vi "9048_main.vi"() -> ()   [LabVIEW 2023]
uses:
  JSON Command.ctl
  Action.ctl
  <vilib>/FPGAPlugInAG/cRIO-9048/niLvFpga_Open_cRIO-9048.vi
  <vilib>/rvi/interface/common/dynamic/niFpgaDynamicAddResources.vi
  <vilib>/Utility/error.llb/Error Cluster From Error Code.vi
  <vilib>/rvi/errors/niLvFpgaAdjustHostInterfaceError.vi
  <vilib>/rvi/interface/common/niFpgaWaitOnOcc.vi
  <vilib>/FPGAPlugInAG/Dynamic/niLvFpga_Run_Dynamic.vi
  <vilib>/FPGAPlugInAG/Dynamic/niLvFpga_Close_Dynamic.vi
  <vilib>/rvi/interface/nirviOpenFPGA/nirviOpenFPGA.xnode
  FPGA Bitfiles/cryosimcontrolsy_FPGATarget_targetmainmem_OolXwFFypuY.lvbitx
  target_main_mem.vi
  <vilib>/rvi/interface/nirviReadWriteControl/nirviReadWriteControl.xnode
  <vilib>/rvi/interface/nirviMethod/nirviMethod.xnode
  <vilib>/rvi/interface/nirviCloseFPGA/nirviCloseFPGA.xnode
  <vilib>/FPGAPlugInAG/Dynamic/niLvFpga_ConfigureFifo_Dynamic.vi
  <vilib>/rvi/errors/niLvFpgaMergeErrorWithErrorCode.vi
  <vilib>/FPGAPlugInAG/Dynamic/niLvFpga_WriteFifo_Dynamic.vi
  NiFpgaLv.dll
  <vilib>/rvi/interface/Simulation/niFpgaSimulationCallBeginRW.vi
  <vilib>/FPGAPlugInAG/Dynamic/niLvFpga_ReadFifo_Dynamic.vi
  <vilib>/FPGAPlugInAG/Dynamic/niLvFpga_StopFifo_Dynamic.vi
  LabView workspace/CoboltLaserDriver.lvlib
panel:
  in  "Stop VI":bool
  out "FPGA VI Reference Out":refnum<k20>
  out "Abort":bool
  out "remote port":u16
  out "remote address":string
  in  "Send PORT":u16=7704
  out "From Client:":string
  out "RAW JSON":T1
  out "ACK sent":string
  in  "FPGA Status Update Loop Time (uSec)":u32=1000
  out "UDP Sent":string
  in  "Event":string
  in  "FPGA Status":string
  in  "Receive PORT":u16=7705
  in  "UDP Address (IP)":string="169.254.31.168"
  out "Digitals":u8
  out "Analogue Line 2":u8
  out "Analogue Line 1":u8
  out "Analogue Line 0":u8
  out "408 Violet Toggle":bool
  in  "Analogue Line 6":u32=20
  out "Laser Port":refnum<visa-resource-name>
  out "Laser Response OK":bool=TRUE
  out "488 Blue Toggle":bool
  out "532 Red Toggle":bool
  out "638 Green Toggle":bool
  in  "Analogue Line 5":u32=20
  in  "Analogue Line 4":u32=20
  in  "Analogue Line 3":u32=20
  in  "Digitals Action Table":T2[](array[typedef])
  in  "Analogue 2 Action Table":T2[](array[typedef])
  in  "Analogue 1 Action Table":T2[](array[typedef])
  in  "Analogue 0 Action Table":T2[](array[typedef])
  out "Tick Ref":u32
  out "Addr Digitals":u32
  out "repDuration (ms)":u64
  out "numReps":u64
  out "From sendStartStopIndexes":u64[](array[numeric])
  out "Addr Analogue 1":u32
  out "Addr Analogue 2":u32
  out "Addr Analogue 0":u32
  in  "att 6":fxp<+/-,20,5> format="%#.3f"
  in  "att 7":fxp<+/-,20,5> format="%#.3f"
  in  "att 5":fxp<+/-,20,5> format="%#.3f"
  in  "att 4":fxp<+/-,20,5> format="%#.3f"
  in  "att 3":fxp<+/-,20,5> format="%#.3f"
  in  "att 2":fxp<+/-,20,5> format="%#.3f"
  in  "att 1":fxp<+/-,20,5> format="%#.3f"
  in  "Vps 5":fxp<+/-,20,5>
  in  "Vps 4":fxp<+/-,20,5>
  in  "Vps 2":fxp<+/-,20,5>
  in  "Vps 6":fxp<+/-,20,5>
  in  "Vps 3":fxp<+/-,20,5>
  in  "Vps 1":fxp<+/-,20,5>
  # "TCP Communication"
  # "UDP Communication"
  # "FPGA: Angle, Phase, and Color"
  # "FPGA: Laser On/Off and Power Control"
  # "Action Tables & Experiment Logging"
  # "Experiment Execution Trace"
  # "FPGA: Direct Set Analogue 1"
  # "FPGA: Direct Set Analogue 2"
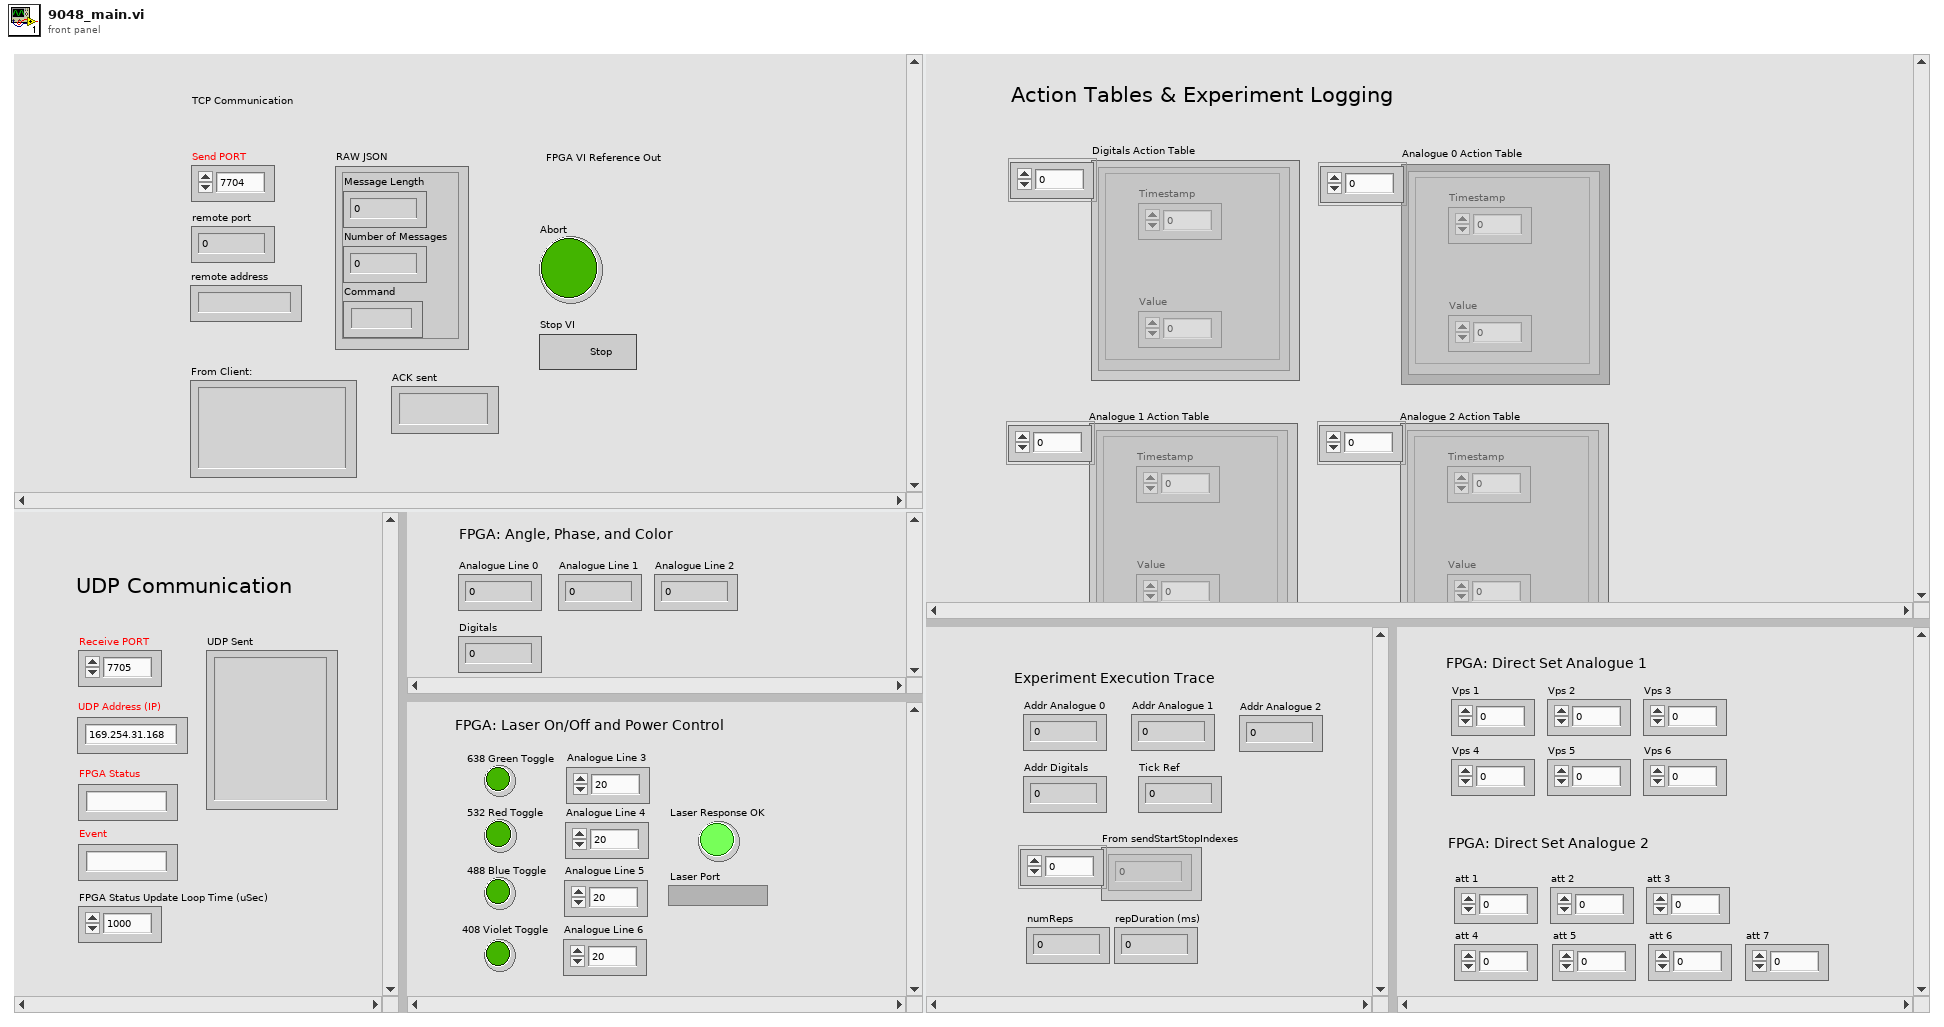
[diagram p1: front panel]
types:
  T1 = typedef "JSON Command.ctl" = cluster{"Message Length":i32, "Number of Messages":i32, "Command":string}
  T2 = typedef "Action.ctl" = cluster{"Timestamp":u32, "Value":u32}
  T3 = cluster{"Digital 0":bool, "Digital 1":bool, "Digital 2":bool}
  T4 = cluster{"Digitals":u8, "Analogue 0":u8, "Analogue 1":u8, "Event":string, "Analogue 2":u8, "Analogue 3":u32, "Analogue 4":u32, "Analogue 5":u32, "Analogue 6":u32}
  T5 = enum16{"Standard", "Buffered", "CRLF", "Immediate"}
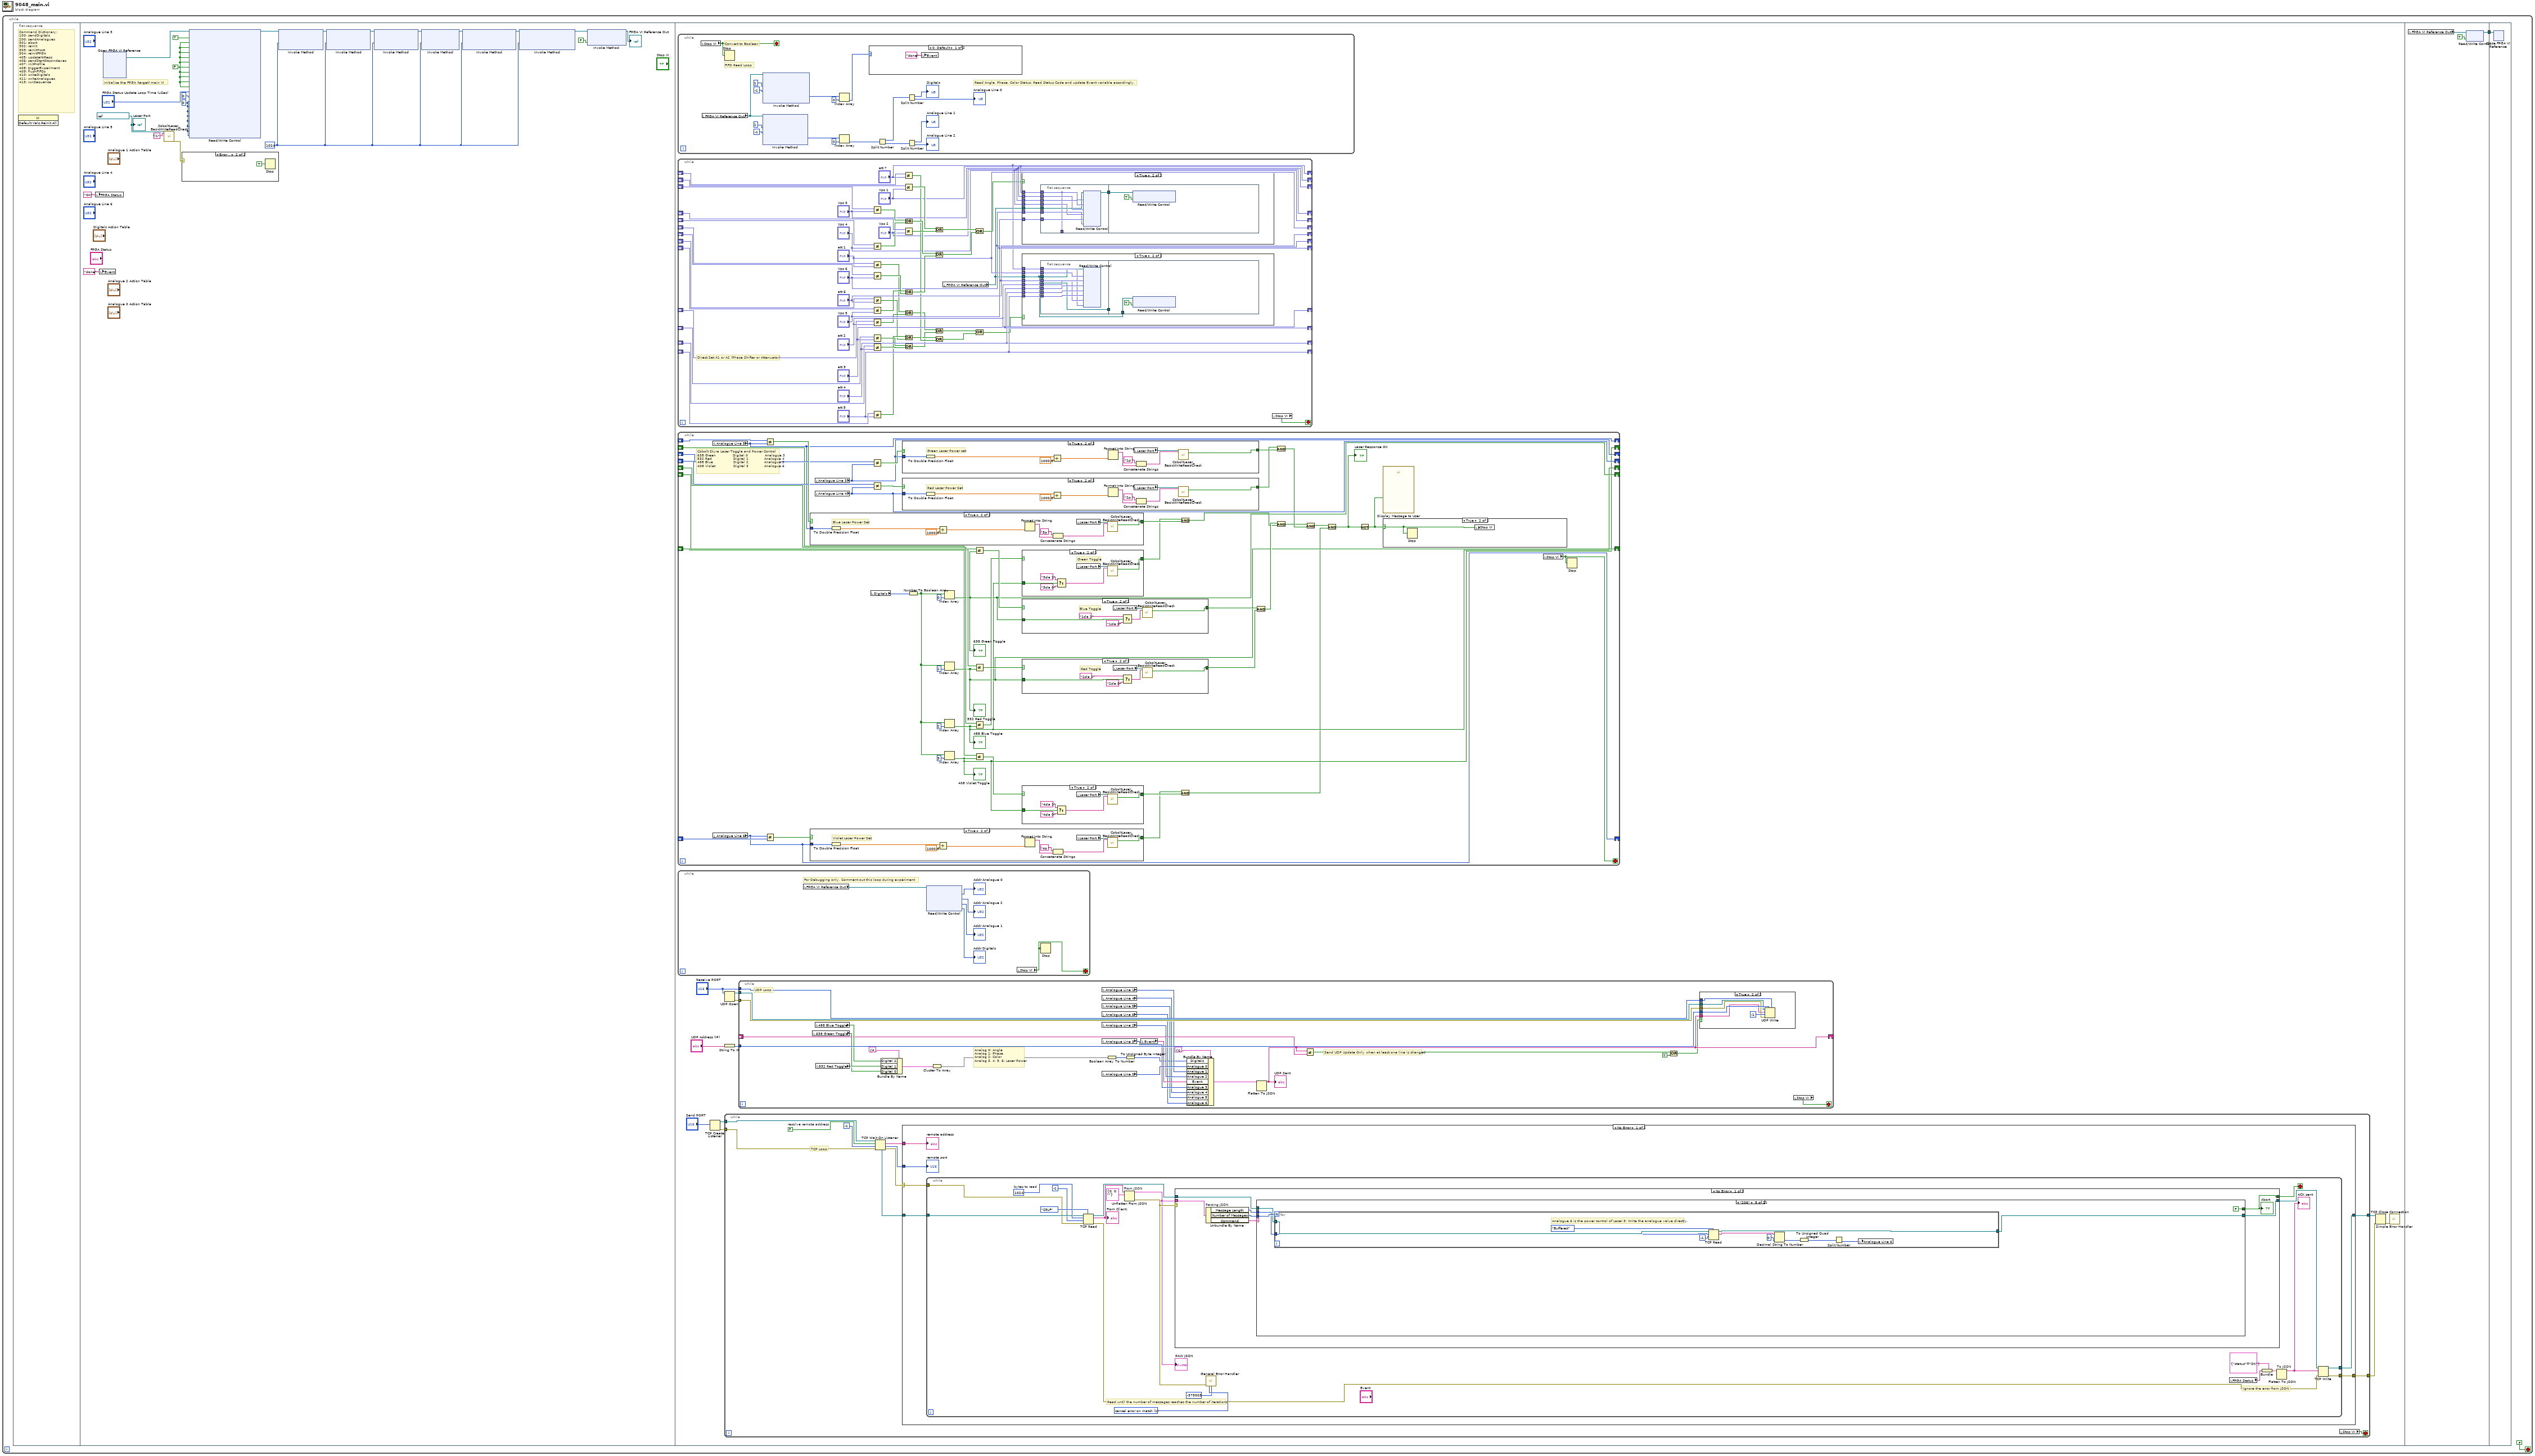
[diagram p0: block diagram]
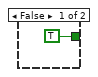
[diagram p5: hidden frame]
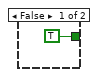
[diagram p6: hidden frame]
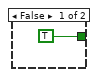
[diagram p8: hidden frame]
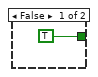
[diagram p9: hidden frame]
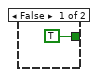
[diagram p10: hidden frame]
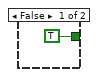
[diagram p11: hidden frame]
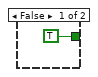
[diagram p12: hidden frame]
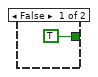
[diagram p13: hidden frame]
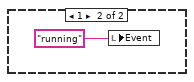
[diagram p14: hidden frame]
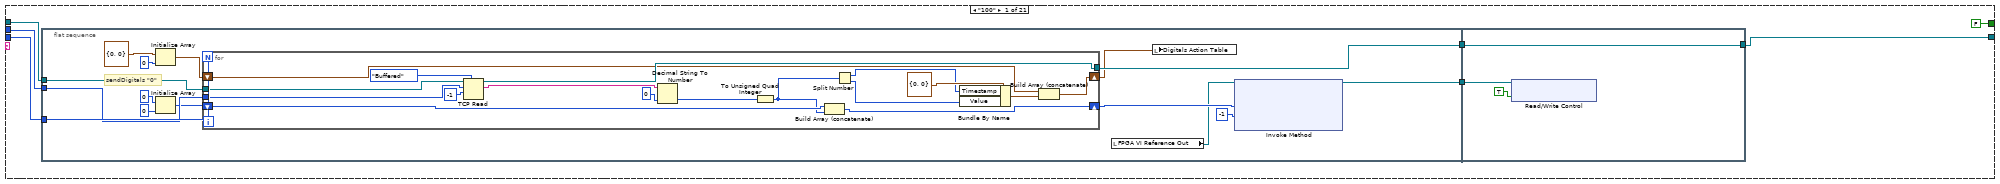
[diagram p16: hidden frame]
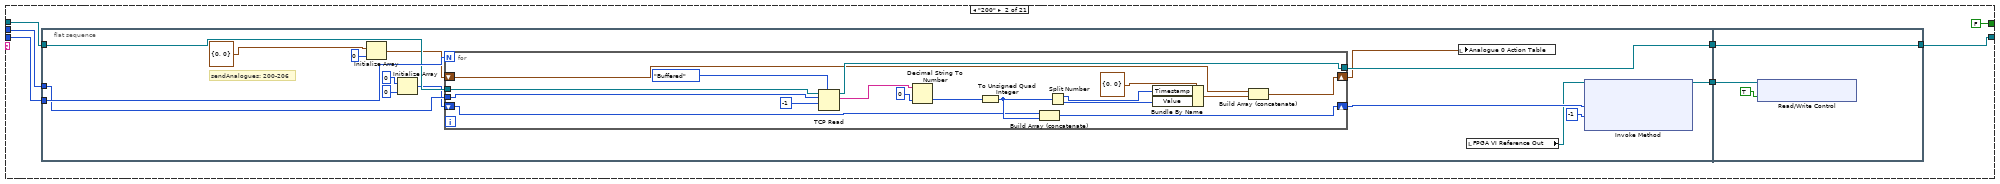
[diagram p17: hidden frame]
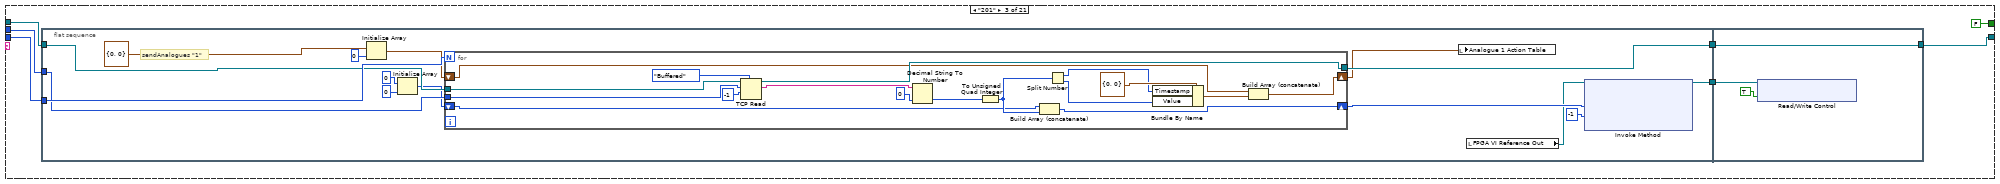
[diagram p18: hidden frame]
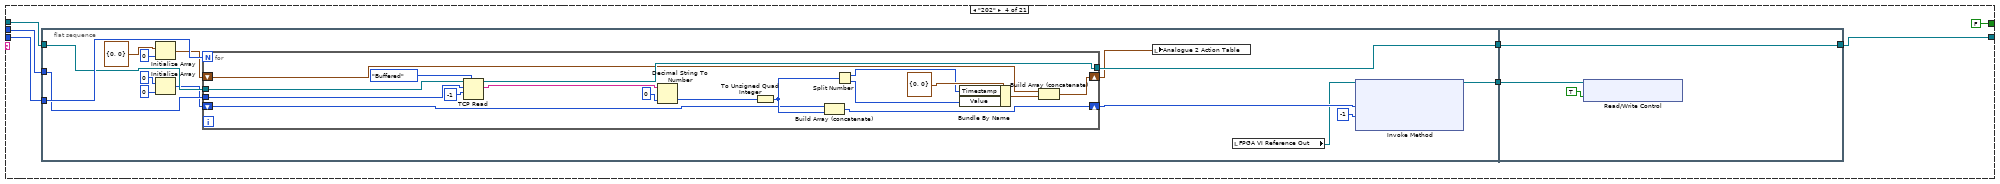
[diagram p19: hidden frame]
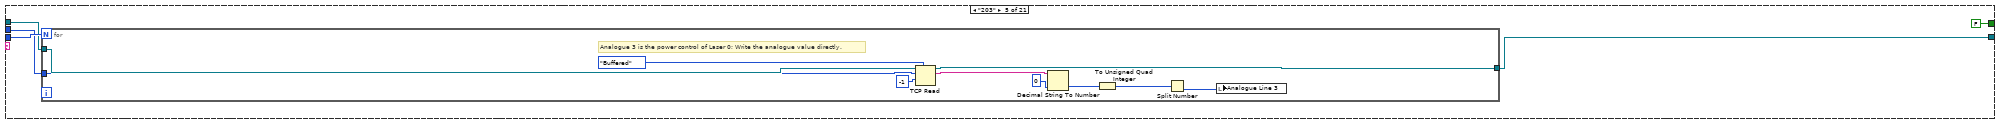
[diagram p20: hidden frame]
diagram:
  n1 = while {
    stop <- FALSE stop-if-true
    n2 = flat-sequence {
      tunnel: [w765] -> w2
      tunnel: w2 -> [w767]
      frame #0 {
        # "Command Dictionary:\n100: sendDigitals\n200: sendAnalogues\n301: abort\n302: reInit\n303: reInitHost\n304: reInitFPGA\n405: updateNrReps\n406: sendStartStopIndexes\n407: initProfile\n408: triggerExperiment\n409: flushFIFOs\n410: writeDigitals\n411: writeAnalogues\n413: runSequence"
        n3 = invoke class="VI" method="Default Vals.Reinit All"() -> ()  [unwired: 3 in, 3 out]
      }
      frame #1 {
        w3 = refnum<visa-resource-name> "ASRL3::INSTR" ("ComPort")
        w9 = u32 0 ("Addr Analogue 0")
        w8 = u32 1024 ("Requested Depth")
        w6 = FALSE ("Action Abort")
        # "Initialize the FPGA (target) main VI"
        n4 = local write "FPGA Status"("OK") -> ()
        n5 = local write "Event"("done") -> ()
        n6 = xnode "Open FPGA VI Reference"() -> ("FPGA VI Reference Out"=w12:refnum<k20>)  [unwired: 2 in, 1 out]
        n7 = call "CoboltLaser_BasicWriteReadCheck.vi"("ComPort"=w3, "Command"="l1") -> ("error out"=w4:errorcluster)  [unwired: 22 in, 3 out]
        n8 = case shown="Error .." w4 {
          frame No Error {
          }
          frame Error {
            n9 = Stop(stop? (T)=TRUE) -> ()
          }
        }
        n10 = xnode "Read/Write Control"("FPGA VI Reference In"=w12, "FPGA Tick Reset"=TRUE, "Abort"=w6, "Load Actions Analogue 0"=w6, "Load Actions Analogue 1"=w6, "Load Actions Analogue 2"=w6, "Load Actions Digitals"=w6, "Flush FIFO"=w6, "Trigger Experiment"=w6, "Set Analogue 0"=w6, "Set Analogue 1"=w6, "Set Analogue 2"=w6, "FPGA Status Update Loop Time (uSec)"="FPGA Status Update Loop Time (uSec)", "Status Code"=u8 0, "Addr Analogue 0"=w9, "Addr Analogue 1"=w9, "Addr Analogue 2"=w9, "Num of Actions Analogue 0"=w9, "Num of Actions Analogue 1"=w9, "Num of Actions Analogue 2"=w9, "Num of Actions Digitals"=w9, "Digitals"=w9) -> ("FPGA VI Reference Out"=w11:refnum<k20>)  [unwired: 1 in, 1 out]
        n11 = xnode "Invoke Method"("FPGA VI Reference In"=w11, "Requested Depth"=w8) -> ("FPGA VI Reference Out"=w22:refnum<k20>)  [unwired: 1 in, 2 out]
        n12 = xnode "Invoke Method"("FPGA VI Reference In"=w22, "Requested Depth"=w8) -> ("FPGA VI Reference Out"=w13:refnum<k20>)  [unwired: 1 in, 2 out]
        n13 = xnode "Invoke Method"("FPGA VI Reference In"=w13, "Requested Depth"=w8) -> ("FPGA VI Reference Out"=w21:refnum<k20>)  [unwired: 1 in, 2 out]
        n14 = xnode "Invoke Method"("FPGA VI Reference In"=w21, "Requested Depth"=w8) -> ("FPGA VI Reference Out"=w20:refnum<k20>)  [unwired: 1 in, 2 out]
        n15 = xnode "Invoke Method"("FPGA VI Reference In"=w20, "Requested Depth"=w8) -> ("FPGA VI Reference Out"=w19:refnum<k20>)  [unwired: 1 in, 2 out]
        n16 = xnode "Invoke Method"("FPGA VI Reference In"=w19, "Requested Depth"=w8) -> ("FPGA VI Reference Out"=w10:refnum<k20>)  [unwired: 1 in, 2 out]
        n17 = xnode "Invoke Method"("FPGA VI Reference In"=w10, "Wait Until Done (F)"=FALSE) -> ("FPGA VI Reference Out"=→"FPGA VI Reference Out":refnum<k20>)  [unwired: 1 in, 1 out]
        "Laser Port" <- w3
      }
      frame #2 {
        n18 = while {
          stop <- w248 stop-if-true
          # "Read Angle, Phase, Color Status; Read Status Code and update Event variable accordingly."
          # "FIFO Read Loop"
          # "Convert to Boolean"
          n19 = local read "Stop VI"() -> (w248:bool)
          n20 = local read "FPGA VI Reference Out"() -> (w249:refnum<k20>)
          n21 = Stop(stop? (T)=w248) -> ()
          n22 = xnode "Invoke Method"("FPGA VI Reference In"=w249, "Number of Elements"=u32 1, "Timeout (ms)"=-1) -> ("Data"=w253:u8[])  [unwired: 1 in, 3 out]
          n23 = xnode "Invoke Method"("FPGA VI Reference In"=w249, "Number of Elements"=u32 1, "Timeout (ms)"=-1) -> ("Data"=w262:u32[])  [unwired: 1 in, 3 out]
          n24 = Index Array(array=w253, index=0) -> (element=w254:u8)
          n25 = Index Array(array=w262, index=0) -> (element=w260:u32)
          n26 = case shown="0, Default" w254 {
            frame 0, Default {
              n27 = local write "Event"("done") -> ()
            }
            frame 1 {
              n28 = local write "Event"("running") -> ()
            }
          }
          n29 = Split Number(x=w260) -> (hi(x)=w259:u16, lo(x)=w258:u16)
          n30 = Split Number(x=w259) -> (hi(x)=→"Digitals":u8, lo(x)=→"Analogue Line 0":u8)
          n31 = Split Number(x=w258) -> (hi(x)=→"Analogue Line 1":u8, lo(x)=→"Analogue Line 2":u8)
        }
        n32 = while {
          shift-right: ["Vps 3"] -> _
          shift-left: _ -> [w85]
          shift-right: ["Vps 4"] -> _
          shift-left: _ -> [w84]
          shift-right: ["Vps 2"] -> _
          shift-left: _ -> [w86]
          shift-right: ["Vps 6"] -> _
          shift-left: _ -> [w82]
          shift-right: ["Vps 5"] -> _
          shift-left: _ -> [w83]
          shift-right: ["Vps 1"] -> _
          shift-left: _ -> [w87]
          shift-right: ["att 1"] -> _
          shift-left: _ -> [w67]
          shift-right: ["att 2"] -> _
          shift-left: _ -> [w66]
          shift-right: ["att 3"] -> _
          shift-left: _ -> [w65]
          shift-right: ["att 4"] -> _
          shift-left: _ -> [w64]
          shift-right: ["att 5"] -> _
          shift-left: _ -> [w63]
          shift-right: ["att 6"] -> _
          shift-left: _ -> [w62]
          shift-right: ["att 7"] -> _
          shift-left: _ -> [w61]
          stop <- w39 stop-if-true
          # "Direct Set A1 or A2 (Phase Shifter or Attenuator)"
          n33 = Not Equal?(x=w85, y="Vps 3") -> (x != y?=w79:bool)
          n34 = Not Equal?(x=w84, y="Vps 4") -> (x != y?=w78:bool)
          n35 = Not Equal?(x=w67, y="att 1") -> (x != y?=w53:bool)
          n36 = Not Equal?(x=w82, y="Vps 6") -> (x != y?=w76:bool)
          n37 = Not Equal?(x=w62, y="att 6") -> (x != y?=w48:bool)
          n38 = Not Equal?(x=w83, y="Vps 5") -> (x != y?=w77:bool)
          n39 = Not Equal?(x=w66, y="att 2") -> (x != y?=w52:bool)
          n40 = Not Equal?(x=w65, y="att 3") -> (x != y?=w51:bool)
          n41 = Not Equal?(x=w64, y="att 4") -> (x != y?=w50:bool)
          n42 = Not Equal?(x=w63, y="att 5") -> (x != y?=w49:bool)
          n43 = Not Equal?(x=w61, y="att 7") -> (x != y?=w47:bool)
          n44 = Not Equal?(x=w87, y="Vps 1") -> (x != y?=w81:bool)
          n45 = Or(x=w79, y=w78) -> (x .or. y?=w74:bool)
          n46 = Not Equal?(x=w86, y="Vps 2") -> (x != y?=w80:bool)
          n47 = Or(x=w77, y=w76) -> (x .or. y?=w73:bool)
          n48 = Or(x=w53, y=w52) -> (x .or. y?=w45:bool)
          n49 = Or(x=w49, y=w48) -> (x .or. y?=w46:bool)
          n50 = Or(x=w51, y=w50) -> (x .or. y?=w44:bool)
          n51 = Or(x=w81, y=w80) -> (x .or. y?=w75:bool)
          n52 = Or(x=w74, y=w73) -> (x .or. y?=w72:bool)
          n53 = Or(x=w45, y=w44) -> (x .or. y?=w42:bool)
          n54 = Or(x=w46, y=w47) -> (x .or. y?=w43:bool)
          n55 = local read "FPGA VI Reference Out"() -> (w40:refnum<k20>)
          n56 = Or(x=w75, y=w72) -> (x .or. y?=w36:bool)
          n57 = Or(x=w42, y=w43) -> (x .or. y?=w41:bool)
          n58 = case shown="True" w36 {
            tunnel: w40 -> [_ w109]
            tunnel: "Vps 1" -> [_ w108]
            tunnel: "Vps 2" -> [_ w114]
            tunnel: "Vps 3" -> [_ w113]
            tunnel: "Vps 4" -> [_ w112]
            tunnel: "Vps 5" -> [_ w111]
            tunnel: "Vps 6" -> [_ w110]
            frame False {
            }
            frame True {
              n59 = flat-sequence {
                tunnel: w109 -> [w117]
                tunnel: w110 -> [w118]
                tunnel: w111 -> [w119]
                tunnel: w112 -> [w120]
                tunnel: w113 -> [w121]
                tunnel: w114 -> [w122]
                tunnel: w108 -> [w115]
                tunnel: [w116] -> w107
                tunnel: [w115] -> _
                tunnel: w107 -> [w123]
                frame #0 {
                  n60 = xnode "Read/Write Control"("FPGA VI Reference In"=w117, "Vps1"=w115, "Vps2"=w122, "Vps3"=w121, "Vps4"=w120, "Vps5"=w119, "Vps6"=w118) -> ("FPGA VI Reference Out"=w116:refnum<k20>)  [unwired: 1 in, 1 out]
                }
                frame #1 {
                  n61 = xnode "Read/Write Control"("FPGA VI Reference In"=w123, "Direct Set Analogue 1"=TRUE) -> ()  [unwired: 1 in, 2 out]
                }
              }
            }
          }
          n62 = case shown="True" w41 {
            tunnel: "att 2" -> [_ w95]
            tunnel: "att 1" -> [_ w96]
            tunnel: "att 3" -> [_ w94]
            tunnel: "att 4" -> [_ w93]
            tunnel: "att 5" -> [_ w92]
            tunnel: "att 6" -> [_ w91]
            tunnel: "att 7" -> [_ w90]
            tunnel: w40 -> [_ w88]
            frame False {
            }
            frame True {
              n63 = flat-sequence {
                tunnel: w88 -> [w97]
                tunnel: w90 -> [w98]
                tunnel: w91 -> [w99]
                tunnel: w92 -> [w100]
                tunnel: w93 -> [w101]
                tunnel: w94 -> [w102]
                tunnel: w95 -> [w103]
                tunnel: w96 -> [w104]
                tunnel: [w97] -> w89
                tunnel: w89 -> [_]
                tunnel: w88 -> [w106]
                frame #0 {
                  n64 = xnode "Read/Write Control"("FPGA VI Reference In"=w97, "att1"=w104, "att2"=w103, "att3"=w102, "att4"=w101, "att5"=w100, "att6"=w99, "att7"=w98) -> ()  [unwired: 1 in, 2 out]
                }
                frame #1 {
                  n65 = xnode "Read/Write Control"("FPGA VI Reference In"=w106, "Direct Set Analogue 2"=TRUE) -> ()  [unwired: 1 in, 2 out]
                }
              }
            }
          }
          n66 = local read "Stop VI"() -> (w39:bool)
        }
        n67 = while {
          shift-right: [w141] -> _
          shift-left: _ -> [w171]
          shift-right: [w139] -> _
          shift-left: _ -> [w166]
          shift-right: [w138] -> _
          shift-left: _ -> [w167]
          shift-right: [w159] -> _
          shift-left: _ -> [w162]
          shift-right: [w158] -> _
          shift-left: _ -> [w161]
          shift-right: [w157] -> _
          shift-left: _ -> [w160]
          shift-right: [w132] -> _
          shift-left: _ -> [w135]
          shift-right: [w129] -> _
          shift-left: _ -> [w131]
          stop <- w146 stop-if-true
          # "Cobolt Skyra Laser Toggle and Power Control\n638 Green               Digital 0               Analogue 3\n532 Red                   Digital 1              Analogue 4\n488 Blue                  Digital 2              Analogue 5\n408 Violet                Digital 3              Analogue 6"
          n68 = local read "Analogue Line 5"() -> (w159:u32)
          n69 = local read "Analogue Line 6"() -> (w129:u32)
          n70 = Not Equal?(x=w162, y=w159) -> (x != y?=w165:bool)
          n71 = Not Equal?(x=w129, y=w131) -> (x != y?=w130:bool)
          n72 = case shown="True" w165 {
            tunnel: w159 -> [_ w214]
            tunnel: [TRUE w212] -> w154
            frame False {
            }
            frame True {
              # "Blue Laser Power Set"
              n73 = To Double Precision Float(number=w214) -> (double precision float=w215:dbl)
              n74 = Divide(x=w215, y=1000.0) -> (x/y=w219:dbl)
              n75 = Format Into String(w219) -> (resulting string=w218:string)  [unwired: 3 in, 1 out]
              n76 = Concatenate Strings("3p " ("string"), w218) -> (w213:string)
              n77 = local read "Laser Port"() -> (w211:refnum<visa-resource-name>)
              n78 = call "CoboltLaser_BasicWriteReadCheck.vi"("ComPort"=w211, "Command"=w213) -> ("ResponseOK"=w212:bool)  [unwired: 22 in, 3 out]
            }
          }
          n79 = case shown="True" w130 {
            tunnel: w129 -> [_ w181]
            tunnel: [TRUE ("ResponseOK") w173] -> w128
            frame False {
            }
            frame True {
              # "Violet Laser Power Set"
              n80 = To Double Precision Float(number=w181) -> (double precision float=w179:dbl)
              n81 = Divide(x=w179, y=1000.0) -> (x/y=w178:dbl)
              n82 = Format Into String(w178) -> (resulting string=w177:string)  [unwired: 3 in, 1 out]
              n83 = Concatenate Strings("4p " ("string"), w177) -> (w174:string)
              n84 = local read "Laser Port"() -> (w175:refnum<visa-resource-name>)
              n85 = call "CoboltLaser_BasicWriteReadCheck.vi"("ComPort"=w175, "Command"=w174) -> ("ResponseOK"=w173:bool)  [unwired: 22 in, 3 out]
            }
          }
          n86 = local read "Analogue Line 3"() -> (w157:u32)
          n87 = local read "Analogue Line 4"() -> (w158:u32)
          n88 = local read "Digitals"() -> (w140:u8)
          n89 = Not Equal?(x=w160, y=w157) -> (x != y?=w163:bool)
          n90 = Not Equal?(x=w161, y=w158) -> (x != y?=w164:bool)
          n91 = case shown="True" w163 {
            tunnel: w157 -> [_ w194]
            tunnel: [TRUE w193] -> w151
            frame False {
            }
            frame True {
              # "Green Laser Power set"
              n92 = To Double Precision Float(number=w194) -> (double precision float=w195:dbl)
              n93 = Divide(x=w195, y=1000.0) -> (x/y=w199:dbl)
              n94 = Format Into String(w199) -> (resulting string=w198:string)  [unwired: 3 in, 1 out]
              n95 = local read "Laser Port"() -> (w191:refnum<visa-resource-name>)
              n96 = Concatenate Strings("1p " ("string"), w198) -> (w192:string)
              n97 = call "CoboltLaser_BasicWriteReadCheck.vi"("ComPort"=w191, "Command"=w192) -> ("ResponseOK"=w193:bool)  [unwired: 22 in, 3 out]
            }
          }
          n98 = case shown="True" w164 {
            tunnel: w158 -> [_ w204]
            tunnel: [TRUE w203] -> w152
            frame False {
            }
            frame True {
              # "Red Laser Power Set"
              n99 = To Double Precision Float(number=w204) -> (double precision float=w205:dbl)
              n100 = Divide(x=w205, y=1000.0) -> (x/y=w209:dbl)
              n101 = Format Into String(w209) -> (resulting string=w208:string)  [unwired: 3 in, 1 out]
              n102 = local read "Laser Port"() -> (w201:refnum<visa-resource-name>)
              n103 = Concatenate Strings("2p " ("string"), w208) -> (w202:string)
              n104 = call "CoboltLaser_BasicWriteReadCheck.vi"("ComPort"=w201, "Command"=w202) -> ("ResponseOK"=w203:bool)  [unwired: 22 in, 3 out]
            }
          }
          n105 = Number To Boolean Array(number=w140) -> (Boolean array=w137:bool[])
          n106 = Index Array(array=w137, index=0) -> (element=w141:bool)
          "638 Green Toggle" <- w141
          n107 = Index Array(array=w137, index=1) -> (element=w139:bool)
          "532 Red Toggle" <- w139
          n108 = Index Array(array=w137, index=2) -> (element=w138:bool)
          "488 Blue Toggle" <- w138
          n109 = Index Array(array=w137, index=3) -> (element=w132:bool)
          "408 Violet Toggle" <- w132
          n110 = Not Equal?(x=w171, y=w141) -> (x != y?=w170:bool)
          n111 = Not Equal?(x=w166, y=w139) -> (x != y?=w169:bool)
          n112 = Not Equal?(x=w167, y=w138) -> (x != y?=w168:bool)
          n113 = Not Equal?(x=w135, y=w132) -> (x != y?=w134:bool)
          n114 = case shown="True" w168 {
            tunnel: w138 -> [_ w224]
            tunnel: [TRUE w222] -> w153
            frame False {
            }
            frame True {
              # "Green Toggle"
              n115 = Select(t="3sla 1", s=w224, f="3sla 0") -> (s? t:f=w223:string)
              n116 = local read "Laser Port"() -> (w221:refnum<visa-resource-name>)
              n117 = call "CoboltLaser_BasicWriteReadCheck.vi"("ComPort"=w221, "Command"=w223) -> ("ResponseOK"=w222:bool)  [unwired: 22 in, 3 out]
            }
          }
          n118 = case shown="True" w170 {
            tunnel: w141 -> [_ w238]
            tunnel: [TRUE w236] -> w156
            frame False {
            }
            frame True {
              # "Blue Toggle"
              n119 = local read "Laser Port"() -> (w235:refnum<visa-resource-name>)
              n120 = Select(t="1sla 1", s=w238, f="1sla 0") -> (s? t:f=w237:string)
              n121 = call "CoboltLaser_BasicWriteReadCheck.vi"("ComPort"=w235, "Command"=w237) -> ("ResponseOK"=w236:bool)  [unwired: 22 in, 3 out]
            }
          }
          n122 = case shown="True" w169 {
            tunnel: w139 -> [_ w230]
            tunnel: [TRUE w229] -> w155
            frame False {
            }
            frame True {
              # "Red Toggle"
              n123 = local read "Laser Port"() -> (w228:refnum<visa-resource-name>)
              n124 = Select(t="2sla 1", s=w230, f="2sla 0") -> (s? t:f=w231:string)
              n125 = call "CoboltLaser_BasicWriteReadCheck.vi"("ComPort"=w228, "Command"=w231) -> ("ResponseOK"=w229:bool)  [unwired: 22 in, 3 out]
            }
          }
          n126 = case shown="True" w134 {
            tunnel: [TRUE ("ResponseOK") w184] -> w133
            tunnel: w132 -> [_ w183]
            frame False {
            }
            frame True {
              n127 = Select(t="4sla 1", s=w183, f="4sla 0") -> (s? t:f=w186:string)
              n128 = local read "Laser Port"() -> (w185:refnum<visa-resource-name>)
              n129 = call "CoboltLaser_BasicWriteReadCheck.vi"("ComPort"=w185, "Command"=w186) -> ("ResponseOK"=w184:bool)  [unwired: 22 in, 3 out]
            }
          }
          n130 = And(x=w153, y=w154) -> (x .and. y?=w149:bool)
          n131 = And(x=w128, y=w133) -> (x .and. y?=w126:bool)
          n132 = And(x=w156, y=w155) -> (x .and. y?=w150:bool)
          n133 = And(x=w152, y=w151) -> (x .and. y?=w148:bool)
          n134 = And(x=w150, y=w149) -> (x .and. y?=w147:bool)
          n135 = And(x=w147, y=w148) -> (x .and. y?=w127:bool)
          n136 = And(x=w127, y=w126) -> (x .and. y?=w125:bool)
          "Laser Response OK" <- w125
          n137 = Not(x=w125) -> (.not. x?=w145:bool)
          n138 = call "Display Message to User"("Enable"=w145) -> ()  [unwired: 9 in, 2 out]
          n139 = case shown="True" w145 {
            selector: w145 -> [_ w189]
            frame False {
            }
            frame True {
              n140 = Stop(stop? (T)=w189) -> ()
              n141 = local write "Stop VI"(w189) -> ()
            }
          }
          n142 = local read "Stop VI"() -> (w146:bool)
          n143 = Stop(stop? (T)=w146) -> ()
        }
        n144 = while {
          stop <- w242 stop-if-true
          # "For Debugging only. Comment out this loop during experiment"
          n145 = local read "FPGA VI Reference Out"() -> (w243:refnum<k20>)
          n146 = xnode "Read/Write Control"("FPGA VI Reference In"=w243) -> ("Addr Analogue 0"=→"Addr Analogue 0":u32, "Addr Analogue 2"=→"Addr Analogue 2":u32, "Addr Analogue 1"=→"Addr Analogue 1":u32, "Addr Digitals"=→"Addr Digitals":u32)  [unwired: 1 in, 2 out]
          n147 = local read "Stop VI"() -> (w242:bool)
          n148 = Stop(stop? (T)=w242) -> ()
        }
        n149 = TCP Create Listener(10:"Send PORT") -> (0:w33:errorcluster, 3:w32:refnum<k5>)  [unwired: 4 in, 1 out]
        n150 = UDP Open(11:"Receive PORT") -> (port=w27:refnum<k16>, 0:w29:errorcluster)  [unwired: 4 in, 1 out]
        n151 = String To IP(1:"UDP Address (IP)") -> (0:w26:u32)
        n152 = while {
          tunnel: w32 -> [w311]
          tunnel: w33 -> [w310]
          tunnel: [w309] -> w34
          tunnel: [w308] -> w35
          stop <- w301 stop-if-true
          w305 = FALSE  # resolve remote address
          # "TCP Loop"
          n153 = TCP Wait On Listener(8:w310, 9:-1 ("timeout ms (wait forever: -1)"), 10:w305, 11:w311) -> (0:w306:errorcluster, 1:w303:u16, 2:w304:string, 4:w302:refnum<k5>)  [unwired: 1 out]
          n154 = case shown="No Error" w306 {
            selector: w306 -> [w314 w762]
            tunnel: w302 -> [w317 w763]
            tunnel: [w316 w762] -> w309
            tunnel: [w315 w763] -> w308
            tunnel: w304 -> [w312 _]
            tunnel: w303 -> [w313 _]
            frame No Error {
              n155 = while {
                tunnel: w314 -> [w328]
                tunnel: [w330] -> w316
                tunnel: w317 -> [w331]
                tunnel: [w329] -> w315
                stop <- w322 stop-if-true
                w326 = 1 items=["no exception", "cancel error on match", "set error on match"] ("[exception action] (none:0)")
                w337 = 1024  # bytes to read
                # "Ignore the error from JSON"
                # "Read until the number of messages reaches the number of iterations"
                n156 = TCP Read(connection ID=w331, bytes to read=w337, error in (no error)=w328, 7:T5."CRLF" ("mode (standard)"), 9:-1 ("timeout ms (25000)")) -> (connection ID out=w320:refnum<k5>, data out=w334:string, error out=w338:errorcluster)
                "From Client:" <- w334
                n157 = Unflatten From JSON "From JSON"(JSON string=w334, type and defaults=T1 {"Message Length"=0, "Number of Messages"=0, "Command"=""} ("JSON Command")) -> (value=w323:T1, error out=w324:errorcluster)  [unwired: 5 in]
                "RAW JSON" <- w323
                n158 = case shown="No Error" w324 {
                  tunnel: w323 -> [w345 _]
                  tunnel: [w343 TRUE] -> w322
                  tunnel: w320 -> [w341 w760]
                  tunnel: [w340 w760] -> w319
                  frame No Error {
                    n159 = Unbundle By Name "Parsing JSON"(w345) -> ("Message Length"=w339:i32, "Number of Messages"=w342:i32, "Command"=w344:string)
                    n160 = case shown="\"206\"" w344 {
                      tunnel: [FALSE FALSE FALSE FALSE FALSE FALSE FALSE FALSE FALSE FALSE FALSE FALSE FALSE FALSE FALSE FALSE FALSE FALSE FALSE FALSE TRUE] -> w343
                      tunnel: w342 -> [w351 w393 w436 w477 w517 w532 w547 w562 _ _ _ _ _ w608 w631 _ _ _ _ _ _]
                      tunnel: w341 -> [w350 w392 w434 w476 w516 w531 w546 w561 w577 w579 w581 w584 w600 w609 w633 w647 w666 w688 w703 w756 w759]
                      tunnel: [w349 w391 w433 w474 w514 w529 w544 w559 w577 w579 w581 w584 w600 w602 w622 w647 w666 w687 w694 w756 w759] -> w340
                      tunnel: w339 -> [w348 w390 w432 w475 w515 w530 w545 w560 _ _ _ _ _ w607 w632 _ _ w685 w699 _ _]
                      frame "100" {
                        n161 = flat-sequence {
                          tunnel: w351 -> [w367]
                          tunnel: w350 -> [w366]
                          tunnel: w348 -> [w364]
                          tunnel: [w365] -> w347
                          tunnel: [w353] -> w346
                          tunnel: [w387] -> w349
                          tunnel: w347 -> [w387]
                          tunnel: w346 -> [w386]
                          frame #0 {
                            # "sendDigitals \"0\""
                            n162 = Initialize Array(T2 {"Timestamp"=0, "Value"=0} ("Action"), 0 ("dimension size")) -> (w359:T2[])
                            n163 = Initialize Array(u64 0 ("element"), 0 ("dimension size")) -> (w358:u64[])
                            n164 = for {
                              N: w367 -> [_]
                              tunnel: w366 -> [w383]
                              tunnel: [w382] -> w365
                              tunnel: w364 -> [w381]
                              shift-right: [w369] -> w356
                              shift-left: w358 -> [w371]
                              shift-right: [w372] -> w357
                              shift-left: w359 -> [w374]
                              n165 = TCP Read(connection ID=w383, bytes to read=w381, 7:T5."Buffered" ("mode (standard)"), 9:-1 ("timeout ms (25000)")) -> (connection ID out=w382:refnum<k5>, data out=w378:string)  [unwired: 1 in, 1 out]
                              n166 = Decimal String To Number(string=w378, default (0L)=u64 0 ("default (0 I32)")) -> (number=w379:u64)  [unwired: 1 in, 1 out]
                              n167 = To Unsigned Quad Integer(1:w379) -> (0:w370:u64)
                              n168 = Build Array (concatenate)(w371, w370) -> (w369:u64[])
                              n169 = Split Number(x=w370) -> (hi(x)=w376:u32, lo(x)=w375:u32)
                              n170 = Bundle By Name(cluster=T2 {"Timestamp"=0, "Value"=0} ("Action"), "Timestamp"=w376, "Value"=w375) -> (w373:T2)
                              n171 = Build Array (concatenate)(w374, w373) -> (w372:T2[])
                            }
                            n172 = local read "FPGA VI Reference Out"() -> (w354:refnum<k20>)
                            n173 = local write "Digitals Action Table"(w357) -> ()
                            n174 = xnode "Invoke Method"("FPGA VI Reference In"=w354, "Data"=w356, "Timeout (ms)"=-1) -> ("FPGA VI Reference Out"=w353:refnum<k20>)  [unwired: 1 in, 2 out]
                          }
                          frame #1 {
                            n175 = xnode "Read/Write Control"("FPGA VI Reference In"=w386, "Load Actions Digitals"=TRUE ("Load Actions")) -> ()  [unwired: 1 in, 2 out]
                          }
                        }
                      }
                      frame "200" {
                        n176 = flat-sequence {
                          tunnel: w393 -> [w409]
                          tunnel: w392 -> [w408]
                          tunnel: w390 -> [w406]
                          tunnel: [w407] -> w389
                          tunnel: [w395] -> w388
                          tunnel: [w429] -> w391
                          tunnel: w389 -> [w429]
                          tunnel: w388 -> [w428]
                          frame #0 {
                            # "sendAnalogues: 200-206"
                            n177 = Initialize Array(T2 {"Timestamp"=0, "Value"=0} ("Action"), 0 ("dimension size")) -> (w403:T2[])
                            n178 = Initialize Array(u64 0 ("element"), 0 ("dimension size")) -> (w399:u64[])
                            n179 = for {
                              N: w409 -> [_]
                              tunnel: w408 -> [w425]
                              tunnel: [w423] -> w407
                              tunnel: w406 -> [w422]
                              shift-right: [w413] -> w402
                              shift-left: w403 -> [w418]
                              shift-right: [w410] -> w398
                              shift-left: w399 -> [w411]
                              n180 = TCP Read(connection ID=w425, bytes to read=w422, 7:T5."Buffered" ("mode (standard)"), 9:-1 ("timeout ms (25000)")) -> (connection ID out=w423:refnum<k5>, data out=w420:string)  [unwired: 1 in, 1 out]
                              n181 = Decimal String To Number(string=w420, default (0L)=u64 0) -> (number=w421:u64)  [unwired: 1 in, 1 out]
                              n182 = To Unsigned Quad Integer(1:w421) -> (0:w412:u64)
                              n183 = Build Array (concatenate)(w411, w412) -> (w410:u64[])
                              n184 = Split Number(x=w412) -> (hi(x)=w416:u32, lo(x)=w415:u32)
                              n185 = Bundle By Name(cluster=T2 {"Timestamp"=0, "Value"=0} ("Action"), "Timestamp"=w416, "Value"=w415) -> (w414:T2)
                              n186 = Build Array (concatenate)(w418, w414) -> (w413:T2[])
                            }
                            n187 = local write "Analogue 0 Action Table"(w402) -> ()
                            n188 = local read "FPGA VI Reference Out"() -> (w396:refnum<k20>)
                            n189 = xnode "Invoke Method"("FPGA VI Reference In"=w396, "Data"=w398, "Timeout (ms)"=-1) -> ("FPGA VI Reference Out"=w395:refnum<k20>)  [unwired: 1 in, 2 out]
                          }
                          frame #1 {
                            n190 = xnode "Read/Write Control"("FPGA VI Reference In"=w428, "Load Actions Analogue 0"=TRUE ("Load Actions")) -> ()  [unwired: 1 in, 2 out]
                          }
                        }
                      }
                      frame "201" {
                        n191 = flat-sequence {
                          tunnel: w436 -> [w451]
                          tunnel: w434 -> [w450]
                          tunnel: w432 -> [w448]
                          tunnel: [w449] -> w431
                          tunnel: [w437] -> w430
                          tunnel: [w471] -> w433
                          tunnel: w431 -> [w471]
                          tunnel: w430 -> [w470]
                          frame #0 {
                            # "sendAnalogues \"1\""
                            n192 = Initialize Array(T2 {"Timestamp"=0, "Value"=0} ("Action"), 0 ("dimension size")) -> (w445:T2[])
                            n193 = Initialize Array(u64 0, 0 ("dimension size")) -> (w440:u64[])
                            n194 = for {
                              N: w451 -> [_]
                              tunnel: w450 -> [w468]
                              tunnel: [w467] -> w449
                              tunnel: w448 -> [w466]
                              shift-right: [w457] -> w443
                              shift-left: w445 -> [w458]
                              shift-right: [w454] -> w439
                              shift-left: w440 -> [w455]
                              n195 = TCP Read(connection ID=w468, bytes to read=w466, 7:T5."Buffered" ("mode (standard)"), 9:-1 ("timeout ms (25000)")) -> (connection ID out=w467:refnum<k5>, data out=w463:string)  [unwired: 1 in, 1 out]
                              n196 = Decimal String To Number(string=w463, default (0L)=u64 0 ("default (0 I32)")) -> (number=w462:u64)  [unwired: 1 in, 1 out]
                              n197 = To Unsigned Quad Integer(1:w462) -> (0:w456:u64)
                              n198 = Build Array (concatenate)(w455, w456) -> (w454:u64[])
                              n199 = Split Number(x=w456) -> (hi(x)=w453:u32, lo(x)=w461:u32)
                              n200 = Bundle By Name(cluster=T2 {"Timestamp"=0, "Value"=0} ("Action"), "Timestamp"=w453, "Value"=w461) -> (w459:T2)
                              n201 = Build Array (concatenate)(w458, w459) -> (w457:T2[])
                            }
                            n202 = local write "Analogue 1 Action Table"(w443) -> ()
                            n203 = local read "FPGA VI Reference Out"() -> (w438:refnum<k20>)
                            n204 = xnode "Invoke Method"("FPGA VI Reference In"=w438, "Data"=w439, "Timeout (ms)"=-1) -> ("FPGA VI Reference Out"=w437:refnum<k20>)  [unwired: 1 in, 2 out]
                          }
                          frame #1 {
                            n205 = xnode "Read/Write Control"("FPGA VI Reference In"=w470, "Load Actions Analogue 1"=TRUE ("Load Actions")) -> ()  [unwired: 1 in, 2 out]
                          }
                        }
                      }
                      frame "202" {
                        n206 = flat-sequence {
                          tunnel: w477 -> [w493]
                          tunnel: w476 -> [w488]
                          tunnel: w475 -> [w487]
                          tunnel: [w486] -> w473
                          tunnel: [w480] -> w472
                          tunnel: [w513] -> w474
                          tunnel: w473 -> [w513]
                          tunnel: w472 -> [w512]
                          frame #0 {
                            n207 = Initialize Array(T2 {"Timestamp"=0, "Value"=0} ("Action"), 0 ("dimension size")) -> (w485:T2[])
                            n208 = Initialize Array(u64 0 ("element"), 0 ("dimension size")) -> (w483:u64[])
                            n209 = for {
                              N: w493 -> [_]
                              tunnel: w488 -> [w509]
                              tunnel: w487 -> [w508]
                              tunnel: [w505] -> w486
                              shift-right: [w498] -> w484
                              shift-left: w485 -> [w499]
                              shift-right: [w495] -> w482
                              shift-left: w483 -> [w496]
                              n210 = TCP Read(connection ID=w509, bytes to read=w508, 7:T5."Buffered" ("mode (standard)"), 9:-1 ("timeout ms (25000)")) -> (connection ID out=w505:refnum<k5>, data out=w506:string)  [unwired: 1 in, 1 out]
                              n211 = Decimal String To Number(string=w506, default (0L)=u64 0 ("default (0 I32)")) -> (number=w504:u64)  [unwired: 1 in, 1 out]
                              n212 = To Unsigned Quad Integer(1:w504) -> (0:w497:u64)
                              n213 = Build Array (concatenate)(w496, w497) -> (w495:u64[])
                              n214 = Split Number(x=w497) -> (hi(x)=w502:u32, lo(x)=w501:u32)
                              n215 = Bundle By Name(cluster=T2 {"Timestamp"=0, "Value"=0} ("Action"), "Timestamp"=w502, "Value"=w501) -> (w500:T2)
                              n216 = Build Array (concatenate)(w499, w500) -> (w498:T2[])
                            }
                            n217 = local write "Analogue 2 Action Table"(w484) -> ()
                            n218 = local read "FPGA VI Reference Out"() -> (w479:refnum<k20>)
                            n219 = xnode "Invoke Method"("FPGA VI Reference In"=w479, "Data"=w482, "Timeout (ms)"=-1) -> ("FPGA VI Reference Out"=w480:refnum<k20>)  [unwired: 1 in, 2 out]
                          }
                          frame #1 {
                            n220 = xnode "Read/Write Control"("FPGA VI Reference In"=w512, "Load Actions Analogue 2"=TRUE ("Load Actions")) -> ()  [unwired: 1 in, 2 out]
                          }
                        }
                      }
                      frame "203" {
                        n221 = for {
                          N: w517 -> [_]
                          tunnel: w516 -> [w527]
                          tunnel: w515 -> [w526]
                          tunnel: [w523] -> w514
                          # "Analogue 3 is the power control of Laser 0; Write the analogue value directly."
                          n222 = TCP Read(connection ID=w527, bytes to read=w526, 7:T5."Buffered" ("mode (standard)"), 9:-1 ("timeout ms (25000)")) -> (connection ID out=w523:refnum<k5>, data out=w524:string)  [unwired: 1 in, 1 out]
                          n223 = Decimal String To Number(string=w524, default (0L)=u64 0 ("default (0 I32)")) -> (number=w522:u64)  [unwired: 1 in, 1 out]
                          n224 = To Unsigned Quad Integer(1:w522) -> (0:w521:u64)
                          n225 = Split Number(x=w521) -> (lo(x)=w519:u32)  [unwired: 1 out]
                          n226 = local write "Analogue Line 3"(w519) -> ()
                        }
                      }
                      frame "204" {
                        n227 = for {
                          N: w532 -> [_]
                          tunnel: w531 -> [w542]
                          tunnel: w530 -> [w541]
                          tunnel: [w538] -> w529
                          # "Analogue 4 is the power control of Laser 1; Write the analogue value directly."
                          n228 = TCP Read(connection ID=w542, bytes to read=w541, 7:T5."Buffered" ("mode (standard)"), 9:-1 ("timeout ms (25000)")) -> (connection ID out=w538:refnum<k5>, data out=w539:string)  [unwired: 1 in, 1 out]
                          n229 = Decimal String To Number(string=w539, default (0L)=u64 0 ("default (0 I32)")) -> (number=w537:u64)  [unwired: 1 in, 1 out]
                          n230 = To Unsigned Quad Integer(1:w537) -> (0:w536:u64)
                          n231 = Split Number(x=w536) -> (lo(x)=w534:u32)  [unwired: 1 out]
                          n232 = local write "Analogue Line 4"(w534) -> ()
                        }
                      }
                      frame "205" {
                        n233 = for {
                          N: w547 -> [_]
                          tunnel: w546 -> [w557]
                          tunnel: w545 -> [w556]
                          tunnel: [w553] -> w544
                          # "Analogue 5 is the power control of Laser 2; Write the analogue value directly."
                          n234 = TCP Read(connection ID=w557, bytes to read=w556, 7:T5."Buffered" ("mode (standard)"), 9:-1 ("timeout ms (25000)")) -> (connection ID out=w553:refnum<k5>, data out=w554:string)  [unwired: 1 in, 1 out]
                          n235 = Decimal String To Number(string=w554, default (0L)=u64 0 ("default (0 I32)")) -> (number=w552:u64)  [unwired: 1 in, 1 out]
                          n236 = To Unsigned Quad Integer(1:w552) -> (0:w551:u64)
                          n237 = Split Number(x=w551) -> (lo(x)=w549:u32)  [unwired: 1 out]
                          n238 = local write "Analogue Line 5"(w549) -> ()
                        }
                      }
                      frame "206" {
                        n239 = for {
                          N: w562 -> [_]
                          tunnel: w561 -> [w572]
                          tunnel: w560 -> [w571]
                          tunnel: [w568] -> w559
                          # "Analogue 6 is the power control of Laser 3; Write the analogue value directly."
                          n240 = TCP Read(connection ID=w572, bytes to read=w571, 7:T5."Buffered" ("mode (standard)"), 9:-1 ("timeout ms (25000)")) -> (connection ID out=w568:refnum<k5>, data out=w569:string)  [unwired: 1 in, 1 out]
                          n241 = Decimal String To Number(string=w569, default (0L)=u64 0 ("default (0 I32)")) -> (number=w567:u64)  [unwired: 1 in, 1 out]
                          n242 = To Unsigned Quad Integer(1:w567) -> (0:w566:u64)
                          n243 = Split Number(x=w566) -> (lo(x)=w564:u32)  [unwired: 1 out]
                          n244 = local write "Analogue Line 6"(w564) -> ()
                        }
                      }
                      frame "301" {
                        w575 = u32 0 ("Num of Actions Analogue 0")
                        # "abort"
                        # "abort"
                        n245 = local read "FPGA VI Reference Out"() -> (w576:refnum<k20>)
                        n246 = xnode "Read/Write Control"("FPGA VI Reference In"=w576, "Trigger Experiment"=FALSE, "Num of Actions Analogue 0"=w575, "Num of Actions Analogue 1"=w575, "Num of Actions Analogue 2"=w575, "Num of Actions Digitals"=w575) -> ()  [unwired: 1 in, 2 out]
                      }
                      frame "302" {
                        # "reInit"
                      }
                      frame "303" {
                        # "reInitHost"
                      }
                      frame "304" {
                        # "reInitFPGA"
                        n247 = flat-sequence {
                          tunnel: [w589] -> w583
                          tunnel: w583 -> [w596]
                          frame #0 {
                            w588 = u32 0 ("Addr Analogue 0")
                            w586 = FALSE ("Abort")
                            w587 = TRUE ("FPGA Tick Reset")
                            n248 = local read "FPGA VI Reference Out"() -> (w595:refnum<k20>)
                            n249 = xnode "Read/Write Control"("FPGA VI Reference In"=w595, "FPGA Tick Reset"=w587, "Flush FIFO"=w587, "Load Actions Analogue 0"=w586, "Load Actions Analogue 1"=w586, "Load Actions Analogue 2"=w586, "Load Actions Digitals"=w586, "Abort"=w586, "Set Analogue 0"=w586, "Set Analogue 1"=w586, "Set Analogue 2"=w586, "Trigger Experiment"=w586, "Status Code"=u8 0, "Addr Analogue 0"=w588, "Addr Analogue 1"=w588, "Addr Analogue 2"=w588, "Addr Digitals"=w588, "Num of Actions Digitals"=w588, "Num of Actions Analogue 0"=w588, "Num of Actions Analogue 1"=w588, "Num of Actions Analogue 2"=w588) -> ("FPGA VI Reference Out"=w590:refnum<k20>)  [unwired: 1 in, 1 out]
                            n250 = xnode "Invoke Method"("FPGA VI Reference In"=w590) -> ("FPGA VI Reference Out"=w593:refnum<k20>)  [unwired: 1 in, 1 out]
                            n251 = xnode "Invoke Method"("FPGA VI Reference In"=w593) -> ("FPGA VI Reference Out"=w592:refnum<k20>)  [unwired: 1 in, 1 out]
                            n252 = xnode "Invoke Method"("FPGA VI Reference In"=w592) -> ("FPGA VI Reference Out"=w591:refnum<k20>)  [unwired: 1 in, 1 out]
                            n253 = xnode "Invoke Method"("FPGA VI Reference In"=w591) -> ("FPGA VI Reference Out"=w589:refnum<k20>)  [unwired: 1 in, 1 out]
                          }
                          frame #1 {
                            n254 = while {
                              tunnel: w596 -> [w597]
                              stop <- w598 stop-if-true
                              n255 = xnode "Read/Write Control"("FPGA VI Reference In"=w597) -> ("Flush FIFO"=w599:bool)  [unwired: 1 in, 2 out]
                              n256 = Not(x=w599) -> (.not. x?=w598:bool)
                            }
                          }
                        }
                      }
                      frame "405" {
                        # "updateNrReps"
                      }
                      frame "406" {
                        # "sendStartStopIndexes"
                        n257 = Initialize Array(u64 0 ("element"), 0 ("dimension size")) -> (w604:u64[])
                        n258 = for {
                          N: w608 -> [_]
                          tunnel: w609 -> [w620]
                          tunnel: w607 -> [w619]
                          shift-right: [w612] -> w603
                          shift-left: w604 -> [w615]
                          tunnel: [w611] -> w602
                          n259 = TCP Read(connection ID=w620, bytes to read=w619, 7:T5."Buffered" ("mode (standard)"), 9:-1 ("timeout ms (25000)")) -> (connection ID out=w611:refnum<k5>, data out=w617:string)  [unwired: 1 in, 1 out]
                          n260 = Decimal String To Number(string=w617, default (0L)=u64 0 ("default (0 I32)")) -> (number=w614:u64)  [unwired: 1 in, 1 out]
                          n261 = To Unsigned Quad Integer(1:w614) -> (0:w613:u64)
                          n262 = Build Array (concatenate)(w615, w613) -> (w612:u64[])
                        }
                        "From sendStartStopIndexes" <- w603
                      }
                      frame "407" {
                        # "initProfile"
                        n263 = Initialize Array(u64 0 ("element"), 0 ("dimension size")) -> (w628:u64[])
                        n264 = for {
                          N: w631 -> [_]
                          tunnel: w633 -> [w644]
                          tunnel: w632 -> [w643]
                          shift-right: [w636] -> w627
                          shift-left: w628 -> [w638]
                          tunnel: [w635] -> w622
                          n265 = TCP Read(connection ID=w644, bytes to read=w643, 9:-1 ("timeout ms (25000)")) -> (connection ID out=w635:refnum<k5>, data out=w641:string)  [unwired: 2 in, 1 out]
                          n266 = Decimal String To Number(string=w641, default (0L)=u64 0 ("default (0 I32)")) -> (number=w639:u64)  [unwired: 1 in, 1 out]
                          n267 = To Unsigned Quad Integer(1:w639) -> (0:w637:u64)
                          n268 = Build Array (concatenate)(w638, w637) -> (w636:u64[])
                        }
                        n269 = Index Array(array=w627, index=1) -> (element=→"repDuration (ms)":u64)
                        n270 = Index Array(array=w627, index=0) -> (element=→"numReps":u64)
                      }
                      frame "408" {
                        # "triggerExperiment"
                        n271 = local read "FPGA VI Reference Out"() -> (w646:refnum<k20>)
                        n272 = flat-sequence {
                          tunnel: w646 -> [w649]
                          tunnel: [w651] -> w645
                          tunnel: w645 -> [w664]
                          frame #0 {
                            n273 = while {
                              tunnel: w649 -> [w660]
                              stop <- w659 stop-if-true
                              # "wait until all actions loaded"
                              n274 = xnode "Read/Write Control"("FPGA VI Reference In"=w660) -> ("Load Actions Analogue 0"=w655:bool, "Load Actions Analogue 1"=w654:bool, "Load Actions Analogue 2"=w653:bool, "Load Actions Analogue 2"=w652:bool)  [unwired: 1 in, 2 out]
                              n275 = Or(x=w655, y=w654) -> (x .or. y?=w657:bool)
                              n276 = Or(x=w653, y=w652) -> (x .or. y?=w656:bool)
                              n277 = Or(x=w657, y=w656) -> (x .or. y?=w658:bool)
                              n278 = Not(x=w658) -> (.not. x?=w659:bool)
                            }
                            n279 = xnode "Read/Write Control"("FPGA VI Reference In"=w649, "FPGA Tick Reset"=TRUE) -> ("FPGA VI Reference Out"=w651:refnum<k20>)  [unwired: 1 in, 1 out]
                          }
                          frame #1 {
                            n280 = xnode "Read/Write Control"("FPGA VI Reference In"=w664, "FPGA Tick Reset"=FALSE, "Trigger Experiment"=TRUE ("FPGA Tick Reset")) -> ("Tick Ref"=→"Tick Ref":u32)  [unwired: 1 in, 2 out]
                          }
                        }
                      }
                      frame "409" {
                        # "flushFIFOs"
                        n281 = flat-sequence {
                          tunnel: [w669] -> w665
                          tunnel: w665 -> [w676]
                          frame #0 {
                            w668 = FALSE ("Load Actions")
                            n282 = local read "FPGA VI Reference Out"() -> (w675:refnum<k20>)
                            n283 = xnode "Read/Write Control"("FPGA VI Reference In"=w675, "Flush FIFO"=TRUE, "Load Actions Analogue 0"=w668, "Load Actions Analogue 1"=w668, "Load Actions Analogue 2"=w668, "Load Actions Digitals"=w668, "Set Analogue 0"=w668, "Set Analogue 1"=w668, "Set Analogue 2"=w668) -> ("FPGA VI Reference Out"=w673:refnum<k20>)  [unwired: 1 in, 1 out]
                            n284 = xnode "Invoke Method"("FPGA VI Reference In"=w673) -> ("FPGA VI Reference Out"=w672:refnum<k20>)  [unwired: 1 in, 1 out]
                            n285 = xnode "Invoke Method"("FPGA VI Reference In"=w672) -> ("FPGA VI Reference Out"=w671:refnum<k20>)  [unwired: 1 in, 1 out]
                            n286 = xnode "Invoke Method"("FPGA VI Reference In"=w671) -> ("FPGA VI Reference Out"=w670:refnum<k20>)  [unwired: 1 in, 1 out]
                            n287 = xnode "Invoke Method"("FPGA VI Reference In"=w670) -> ("FPGA VI Reference Out"=w669:refnum<k20>)  [unwired: 1 in, 1 out]
                          }
                          frame #1 {
                            n288 = while {
                              tunnel: w676 -> [w677]
                              stop <- w678 stop-if-true
                              # "wait until FPGA target flushes FIFO"
                              n289 = xnode "Read/Write Control"("FPGA VI Reference In"=w677) -> ("Flush FIFO"=w679:bool)  [unwired: 1 in, 2 out]
                              n290 = Not(x=w679) -> (.not. x?=w678:bool)
                            }
                          }
                        }
                      }
                      frame "410" {
                        # "writeDigitals"
                        n291 = TCP Read(connection ID=w688, bytes to read=w685, 7:T5."Buffered" ("mode (standard)"), 9:-1 ("timeout ms (25000)")) -> (connection ID out=w687:refnum<k5>, data out=w682:string)  [unwired: 1 in, 1 out]
                        n292 = local read "FPGA VI Reference Out"() -> (w681:refnum<k20>)
                        n293 = Decimal String To Number(string=w682, default (0L)=u32 0 ("default (0 I32)")) -> (number=w680:u32)  [unwired: 1 in, 1 out]
                        n294 = xnode "Read/Write Control"("FPGA VI Reference In"=w681, "Digitals"=w680) -> ()  [unwired: 1 in, 2 out]
                      }
                      frame "411" {
                        # "writeAnalogue"
                        n295 = TCP Read(connection ID=w703, bytes to read=w699, 7:T5."Buffered" ("mode (standard)"), 9:-1 ("timeout ms (25000)")) -> (connection ID out=w700:refnum<k5>, data out=w705:string, error out=w697:errorcluster)  [unwired: 1 in]
                        n296 = Decimal String To Number(string=w705, default (0L)=u32 0 ("default (0 I32)")) -> (number=w693:u32)  [unwired: 1 in, 1 out]
                        n297 = TCP Read(connection ID=w700, bytes to read=w699, error in (no error)=w697, 7:T5."Buffered" ("mode (standard)"), 9:-1 ("timeout ms (25000)")) -> (connection ID out=w694:refnum<k5>, data out=w695:string)  [unwired: 1 out]
                        n298 = local read "FPGA VI Reference Out"() -> (w690:refnum<k20>)
                        n299 = Decimal String To Number(string=w695, default (0L)=u32 0 ("default (0 I32)")) -> (number=w691:u32)  [unwired: 1 in, 1 out]
                        n300 = case shown="6" w693 {
                          tunnel: w691 -> [w709 w724 w739 w752 w753 w754 w755 _]
                          tunnel: w690 -> [w710 w725 w740 _ _ _ _ _]
                          frame 0 {
                            n301 = flat-sequence {
                              tunnel: w710 -> [w715]
                              tunnel: w709 -> [w714]
                              tunnel: [w712] -> w708
                              tunnel: [w711] -> w707
                              tunnel: w708 -> [w717]
                              tunnel: w707 -> [w716]
                              frame #0 {
                                n302 = xnode "Read/Write Control"("FPGA VI Reference In"=w715, "Analogue 0"=w714, "Set Analogue 0"=TRUE) -> ("FPGA VI Reference Out"=w712:refnum<k20>, "error out"=w711:errorcluster)  [unwired: 1 in]
                              }
                              frame #1 {
                                n303 = while {
                                tunnel: w717 -> [w721]
                                tunnel: w716 -> [w720]
                                stop <- w718 stop-if-true
                                n304 = xnode "Read/Write Control"("FPGA VI Reference In"=w721, "error in"=w720) -> ("Set Analogue 0"=w719:bool)  [unwired: 2 out]
                                n305 = Not(x=w719) -> (.not. x?=w718:bool)
                                }
                              }
                            }
                          }
                          frame 1 {
                            n306 = flat-sequence {
                              tunnel: w725 -> [w730]
                              tunnel: w724 -> [w729]
                              tunnel: [w727] -> w723
                              tunnel: [w726] -> w722
                              tunnel: w723 -> [w732]
                              tunnel: w722 -> [w731]
                              frame #0 {
                                n307 = xnode "Read/Write Control"("FPGA VI Reference In"=w730, "Analogue 1"=w729, "Set Analogue 1"=TRUE ("Set Analogue 0")) -> ("FPGA VI Reference Out"=w727:refnum<k20>, "error out"=w726:errorcluster)  [unwired: 1 in]
                              }
                              frame #1 {
                                n308 = while {
                                tunnel: w732 -> [w736]
                                tunnel: w731 -> [w735]
                                stop <- w733 stop-if-true
                                n309 = xnode "Read/Write Control"("FPGA VI Reference In"=w736, "error in"=w735) -> ("Set Analogue 1"=w734:bool)  [unwired: 2 out]
                                n310 = Not(x=w734) -> (.not. x?=w733:bool)
                                }
                              }
                            }
                          }
                          frame 2 {
                            n311 = flat-sequence {
                              tunnel: w740 -> [w745]
                              tunnel: w739 -> [w744]
                              tunnel: [w742] -> w738
                              tunnel: [w741] -> w737
                              tunnel: w738 -> [w747]
                              tunnel: w737 -> [w746]
                              frame #0 {
                                n312 = xnode "Read/Write Control"("FPGA VI Reference In"=w745, "Analogue 2"=w744, "Set Analogue 2"=TRUE ("Set Analogue 0")) -> ("FPGA VI Reference Out"=w742:refnum<k20>, "error out"=w741:errorcluster)  [unwired: 1 in]
                              }
                              frame #1 {
                                n313 = while {
                                tunnel: w747 -> [w751]
                                tunnel: w746 -> [w750]
                                stop <- w748 stop-if-true
                                n314 = xnode "Read/Write Control"("FPGA VI Reference In"=w751, "error in"=w750) -> ("Set Analogue 2"=w749:bool)  [unwired: 2 out]
                                n315 = Not(x=w749) -> (.not. x?=w748:bool)
                                }
                              }
                            }
                          }
                          frame 3 {
                            n316 = local write "Analogue Line 3"(w752) -> ()
                          }
                          frame 4 {
                            n317 = local write "Analogue Line 4"(w753) -> ()
                          }
                          frame 5 {
                            n318 = local write "Analogue Line 5"(w754) -> ()
                          }
                          frame 6 {
                            n319 = local write "Analogue Line 6"(w755) -> ()
                          }
                          frame Default {
                          }
                        }
                      }
                      frame "413" {
                        # "runSequence"
                      }
                      frame "666", Default {
                      }
                    }
                    "Abort" <- w343
                  }
                  frame Error {
                  }
                }
                n320 = call <vilib>:"General Error Handler.vi"("error in (no error)"=w324, "[exception action] (none:0)"=w326, "[exception code]"=-375003) -> ()  [unwired: 8 in, 5 out]
                n321 = local read "FPGA Status"() -> (w318:string)
                n322 = Bundle(cluster=cluster{"status":string} {"status"="OK"}, "status"=w318) -> (w335:cluster{"status":string})
                n323 = Flatten To JSON "To JSON"(anything=w335) -> (JSON string=w321:string)  [unwired: 2 in, 1 out]
                "ACK sent" <- w321
                n324 = TCP Write(connection ID=w319, data in=w321, error in (no error)=w338) -> (connection ID out=w329:refnum<k5>, error out=w330:errorcluster)  [unwired: 1 in, 1 out]
              }
              "remote address" <- w312
              "remote port" <- w313
            }
            frame Error {
            }
          }
          n325 = local read "Stop VI"() -> (w301:bool)
        }
        n326 = while {
          tunnel: w26 -> [w294]
          tunnel: w27 -> [w293]
          tunnel: "Receive PORT" -> [w292]
          tunnel: w29 -> [w291]
          shift-right: [w272] -> _
          shift-left: _ -> [w271]
          stop <- w285 stop-if-true
          # "Send UDP Update Only when at least one line is changed"
          # "UDP Loop"
          # "Analog 0: Angle\nAnalog 1: Phase\nAnalog 2: Color\nAnalog 3, 4, 5, 6: Laser Power"
          n327 = local read "638 Green Toggle"() -> (w277:bool)
          n328 = local read "488 Blue Toggle"() -> (w279:bool)
          n329 = local read "532 Red Toggle"() -> (w278:bool)
          n330 = Bundle By Name(cluster=T3 {"Digital 0"=FALSE, "Digital 1"=FALSE, "Digital 2"=FALSE}, "Digital 2"=w279, "Digital 1"=w278, "Digital 0"=w277) -> (w276:T3)
          n331 = Cluster To Array(cluster=w276) -> (array=w275:bool[])
          n332 = local read "Analogue Line 1"() -> (w287:u8)
          n333 = local read "Analogue Line 4"() -> (w283:u32)
          n334 = local read "Analogue Line 5"() -> (w282:u32)
          n335 = local read "Analogue Line 6"() -> (w267:u32)
          n336 = local read "Analogue Line 2"() -> (w286:u8)
          n337 = local read "Analogue Line 3"() -> (w284:u32)
          n338 = local read "Analogue Line 0"() -> (w288:u8)
          n339 = Boolean Array To Number(Boolean array=w275) -> (number=w281:u32)
          n340 = To Unsigned Byte Integer(number=w281) -> (unsigned 8bit integer=w280:u8)
          n341 = local read "Event"() -> (w289:string)
          n342 = Bundle By Name(cluster=T4 {"Digitals"=0, "Analogue 0"=0, "Analogue 1"=0, "Event"="done", "Analogue 2"=0, "Analogue 3"=0, "Analogue 4"=0, "Analogue 5"=0, "Analogue 6"=0}, "Digitals"=w280, "Analogue 0"=w288, "Analogue 1"=w287, "Analogue 2"=w286, "Event"=w289, "Analogue 3"=w284, "Analogue 4"=w283, "Analogue 5"=w282, "Analogue 6"=w267) -> (w273:T4)
          n343 = Flatten To JSON(anything=w273) -> (JSON string=w272:string)  [unwired: 2 in, 1 out]
          "UDP Sent" <- w272
          n344 = Not Equal?(x=w272, y=w271) -> (x != y?=w270:bool)
          n345 = Or(x=w270, y=TRUE) -> (x .or. y?=w269:bool)
          n346 = case shown="True" w269 {
            tunnel: w294 -> [_ w300]
            tunnel: w293 -> [_ w298]
            tunnel: w292 -> [_ w297]
            tunnel: w291 -> [_ w296]
            tunnel: w272 -> [_ w295]
            frame False {
            }
            frame True {
              n347 = UDP Write(address=w300, port or service name=w297, connection ID=w298, data in=w295, 8:w296, 9:-1 ("timeout ms (25000)")) -> ()  [unwired: 2 out]
            }
          }
          n348 = local read "Stop VI"() -> (w285:bool)
        }
        n349 = TCP Close Connection(connection ID=w35, error in (no error)=w34) -> (error out=w30:errorcluster)  [unwired: 1 in, 1 out]
        n350 = call <vilib>:"Simple Error Handler.vi"("error in (no error)"=w30) -> ()  [unwired: 4 in, 5 out]
      }
      frame #3 {
        n351 = local read "FPGA VI Reference Out"() -> (w766:refnum<k20>)
        n352 = xnode "Read/Write Control"("FPGA VI Reference In"=w766, "Abort"=TRUE) -> ("FPGA VI Reference Out"=w765:refnum<k20>)  [unwired: 1 in, 1 out]
      }
      frame #4 {
        n353 = xnode "Close FPGA VI Reference"("FPGA VI Reference In"=w767) -> ()  [unwired: 1 in, 1 out]
      }
    }
  }
